vi "Despence Product.vi"(8 "error in (no error)":errorcluster, 11 "Stock Item":u32) -> (0 "error out":errorcluster)   [LabVIEW 2020, in "Model.lvlib"]
uses:
  Model.lvlib
  Stock/Stock.lvlib
  Display/Display.lvlib
  Money/Money.lvlib
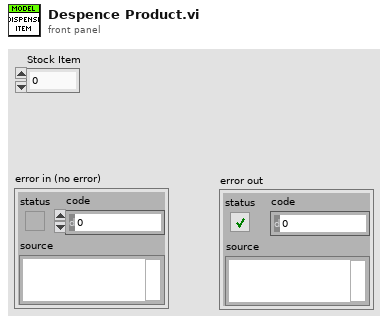
[diagram p1: front panel]
types:
  T1 = typedef "Money.lvlib/Check Funds (Reply Payload)--cluster.ctl" = cluster{"Sufficient Funds":bool, "Check Funds_error":errorcluster, "Balance":u32}
  T2 = typedef "Money.lvlib/Add to Balance (Reply Payload)--cluster.ctl" = cluster{"Add to Balance_error":errorcluster, "New Balance":u32}
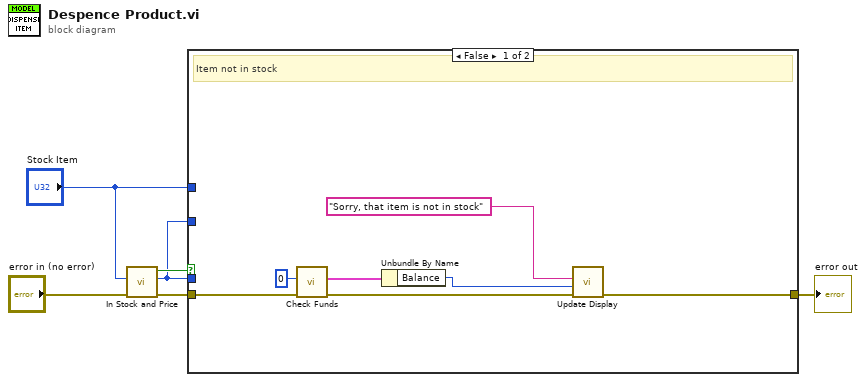
[diagram p0: block diagram]
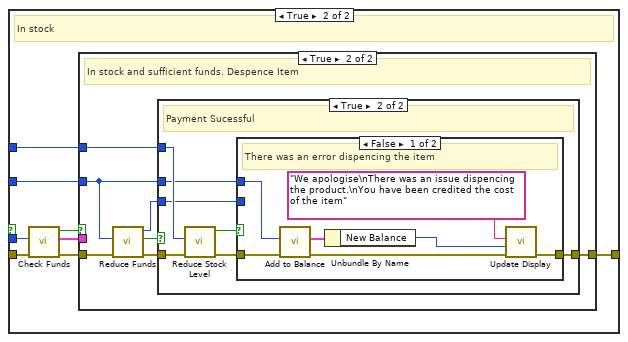
[diagram p2: hidden frame]
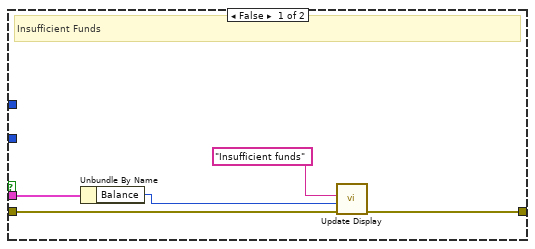
[diagram p3: hidden frame]
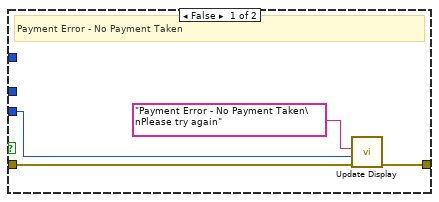
[diagram p4: hidden frame]
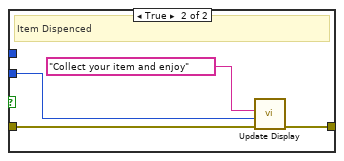
[diagram p5: hidden frame]
diagram:
  n1 = call "In Stock and Price.vi"("error in (no error)"="error in (no error)", "Stock Item"="Stock Item") -> ("error out"=w5:errorcluster, "Price (Pence)"=w4:u32, "In Stock?"=w6:bool)  [unwired: 5 in, 2 out]
  n2 = case shown="False" w6 {
    tunnel: w4 -> [_ w21]
    tunnel: w5 -> [w11 w20]
    tunnel: [w12 w17] -> w2
    tunnel: "Stock Item" -> [_ w16]
    tunnel: w4 -> [_ w15]
    frame False {
      # "Item not in stock"
      n3 = call "Check Funds.vi"("error in (no error)"=w11, "Minimum Amount"=u32 0) -> ("error out"=w10:errorcluster, "Reply Payload"=w9:T1)  [unwired: 6 in, 2 out]
      n4 = Unbundle By Name(w9) -> ("Balance"=w8:u32)
      n5 = call "Update Display.vi"("error in (no error)"=w10, "Balance"=w8, "Message to display"="Sorry, that item is not in stock" ("initial string")) -> ("error out"=w12:errorcluster)  [unwired: 8 in]
    }
    frame True {
      # "In stock"
      n6 = call "Check Funds.vi"("error in (no error)"=w20, "Minimum Amount"=w21) -> ("error out"=w19:errorcluster, "Reply Payload"=w14:T1, "Sufficient Funds"=w18:bool)  [unwired: 6 in, 1 out]
      n7 = case shown="True" w18 {
        tunnel: w19 -> [w24 w32]
        tunnel: [w25 w29] -> w17
        tunnel: w16 -> [_ w33]
        tunnel: w15 -> [_ w27]
        tunnel: w14 -> [w23 _]
        frame False {
          # "Insufficient Funds"
          n8 = Unbundle By Name(w23) -> ("Balance"=w22:u32)
          n9 = call "Update Display.vi"("error in (no error)"=w24, "Balance"=w22, "Message to display"="Insufficient funds" ("initial string")) -> ("error out"=w25:errorcluster)  [unwired: 8 in]
        }
        frame True {
          # "In stock and sufficient funds. Despence Item"
          n10 = call "Reduce Funds.vi"("error in (no error)"=w32, "Reduce Funds"=w27) -> ("error out"=w31:errorcluster, "Sucessful"=w30:bool, "Remaining Balance"=w28:u32)  [unwired: 5 in, 2 out]
          n11 = case shown="True" w30 {
            tunnel: w33 -> [_ w44]
            tunnel: w31 -> [w36 w43]
            tunnel: [w35 w38] -> w29
            tunnel: w28 -> [w34 w40]
            tunnel: w27 -> [_ w39]
            frame False {
              # "Payment Error - No Payment Taken"
              n12 = call "Update Display.vi"("error in (no error)"=w36, "Balance"=w34, "Message to display"="Payment Error - No Payment Taken\nPlease try again" ("initial string")) -> ("error out"=w35:errorcluster)  [unwired: 8 in]
            }
            frame True {
              # "Payment Sucessful"
              n13 = call "Reduce Stock Level.vi"("error in (no error)"=w43, "Product"=w44) -> ("error out"=w42:errorcluster, "Sucessful?"=w41:bool)  [unwired: 6 in, 2 out]
              n14 = case shown="False" w41 {
                tunnel: w42 -> [w49 w54]
                tunnel: w40 -> [_ w52]
                tunnel: w39 -> [w48 _]
                tunnel: [w47 w53] -> w38
                frame False {
                  # "There was an error dispencing the item"
                  n15 = call "Add to Balance.vi"("error in (no error)"=w49, "Balance to add"=w48) -> ("error out"=w50:errorcluster, "Reply Payload"=w46:T2)  [unwired: 7 in, 1 out]
                  n16 = Unbundle By Name(w46) -> ("New Balance"=w45:u32)
                  n17 = call "Update Display.vi"("error in (no error)"=w50, "Balance"=w45, "Message to display"="We apologise\nThere was an issue dispencing the product.\nYou have been credited the cost of the item" ("initial string")) -> ("error out"=w47:errorcluster)  [unwired: 8 in]
                }
                frame True {
                  # "Item Dispenced"
                  n18 = call "Update Display.vi"("error in (no error)"=w54, "Balance"=w52, "Message to display"="Collect your item and enjoy" ("initial string")) -> ("error out"=w53:errorcluster)  [unwired: 8 in]
                }
              }
            }
          }
        }
      }
    }
  }
  "error out" <- w2
